vi "main image(SubVI).vi"(6 "Numeric":i32, 9 "filename  and array":string[](array[string]), 10 "stripped path to folder":path, 11 "Refnum in":T1) -> (3 "Refnum out":T1)   [LabVIEW 2014]
uses:
  <vilib>/vision/Image Controls.llb/IMAQ Image.ctl
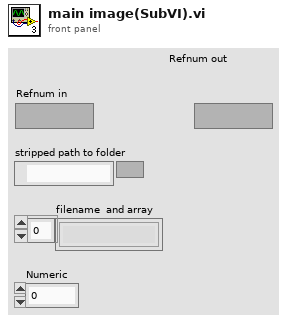
[diagram p1: front panel]
types:
  T1 = typedef "IMAQ Image.ctl" = refnum<image>
  T2 = cluster{"Read Raw File":i32, "File Data Type":u32, "Offset to Data":i32, "Use Min Max":enum32{"Don't use min max", "Use file values", "Use optional values"}, "Optional Min Value":sgl, "Optional Max Value":sgl, "Byte Order":enum32{"Big endian (Motorola)", "Little endian (Intel)"}}
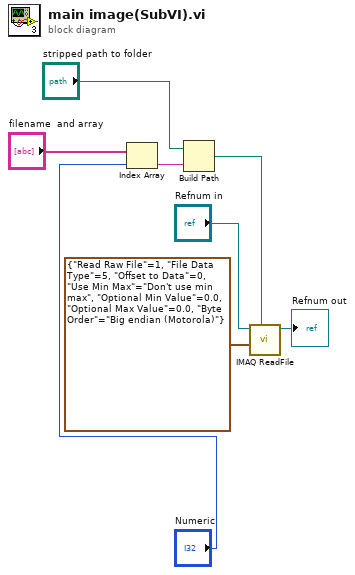
[diagram p0: block diagram]
diagram:
  n1 = Index Array(array="filename  and array", index="Numeric") -> (element=w6:string)
  n2 = Build Path(base path="stripped path to folder", name or relative path=w6) -> (appended path=w4:path)
  n3 = call "IMAQ ReadFile"("File Path"=w4, "File Options"=T2 {"Read Raw File"=1, "File Data Type"=5, "Offset to Data"=0, "Use Min Max"=enum."Don't use min max", "Optional Min Value"=0.0, "Optional Max Value"=0.0, "Byte Order"=enum."Big endian (Motorola)"}, "Image"="Refnum in") -> ("Image Out"=→"Refnum out":T1)  [unwired: 4 in, 4 out]
